vi "DiffDrivePoseEst_BiConsum_VisionCorrect.vi"(9 "Y":T2, 10 "U":T2, 11 "ExtraPassedData":variant) -> (0 "Error":bool, 3 "ExtraReturnedData":variant)   [LabVIEW 2019, in "Trajectory_Library.lvlib"]
doc: "Creates a new LINEAR SYSTEM data cluster with the specified values. \n\n\nInputs: \n - XXX -- XXX.\n\nOutputs:\n - XXX -- XXX."
uses:
  <vilib>/Analysis/Matrix/Datatypes/RealMatrix.ctl
  MatBuilder_Create.vi
  Trajectory_Library.lvlib
  DiffDrivePoseEst_BiFunc_H.vi
  AngleStats_AngleMean_BiFunc.vi
  AngleStats_AngleResidual_BiFunc.vi
  AngleStats_AngleAdd_BiFunc.vi
  <vilib>/Analysis/Matrix/NI_Matrix.lvlib
  MERWE_SCALED_SIGMA_PTS.ctl
  BiFun_Matrix_FUNC_TYPE.ctl
  UNSCENTED_KALMAN_FILTER.ctl
panel:
  in  "Cluster":T5
  # "State Estimate <Statess,1>"
  # "<States, States>"
  # "<States, ?>"
  # "<Statess,  States>"
  # "<Outputs, Outputs>"
  # "<?, 1>"
  # "<?, 1>"
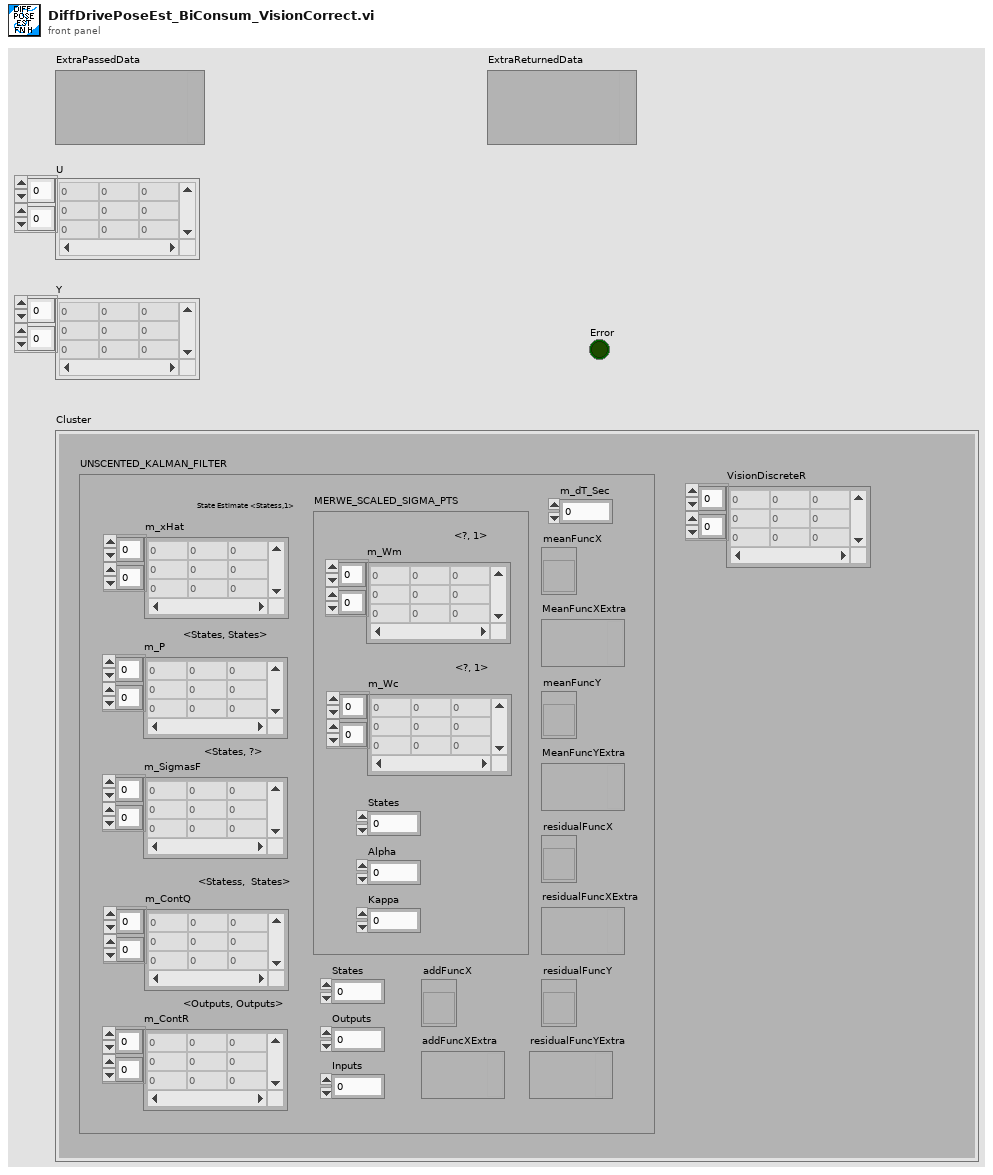
[diagram p1: front panel]
types:
  T1 = typedef "Trajectory_Library.lvlib/UNSCENTED_KALMAN_FILTER.ctl" = cluster{"m_P":T2, "m_xHat":T2, "States":i32, "Outputs":i32, "m_ContR":T2, "m_ContQ":T2, "m_SigmasF":T2, "m_dT_Sec":dbl, "MERWE_SCALED_SIGMA_PTS":T3, "meanFuncX":T4, "meanFuncY":T4, "residualFuncX":T4, "residualFuncY":T4, "addFuncX":T4, "addFuncXExtra":variant, "residualFuncYExtra":variant, "residualFuncXExtra":variant, "MeanFuncYExtra":variant, "MeanFuncXExtra":variant, "Inputs":i32}
  T2 = typedef "NI_Matrix.lvlib/RealMatrix.ctl" = dbl[][]
  T3 = typedef "Trajectory_Library.lvlib/MERWE_SCALED_SIGMA_PTS.ctl" = cluster{"m_Wm":T2, "States":i32, "Alpha":dbl, "m_Wc":T2, "Kappa":i32}
  T4 = typedef "Trajectory_Library.lvlib/BiFun_Matrix_FUNC_TYPE.ctl" = refnum<vi>
  T5 = cluster{"UNSCENTED_KALMAN_FILTER":T1, "VisionDiscreteR":T2}
  T6 = typedef "Trajectory_Library.lvlib/UNSCENTED_KALMAN_CORRECT_FUNC_GROUP.ctl" = cluster{"H_Func":T4, "meanFuncY":T4, "residualFuncY":T4, "residualFuncX":T4, "addFuncX":T4, "H_FuncExtra":variant, "MeanFuncYExtra":variant, "residualFuncYExtra":variant, "residualFuncXExtra":variant, "addFuncXExtra":variant}
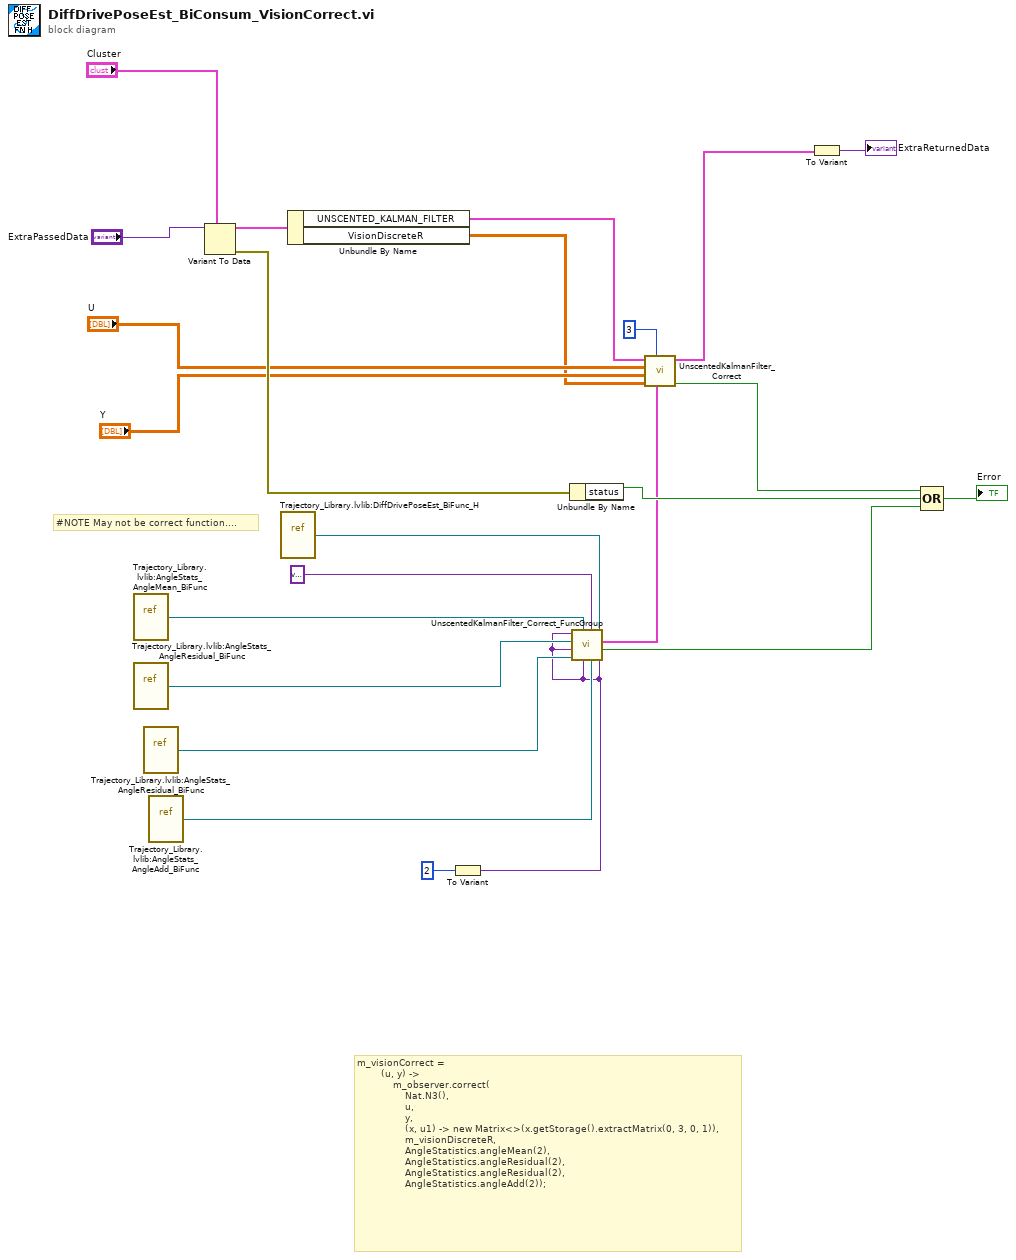
[diagram p0: block diagram]
diagram:
  # "#NOTE May not be correct function...."
  # "m_visionCorrect =\n        (u, y) ->\n            m_observer.correct(\n                Nat.N3(),\n                u,\n                y,\n                (x, u1) -> new Matrix<>(x.getStorage().extractMatrix(0, 3, 0, 1)),\n                m_visionDiscreteR,\n                AngleStatistics.angleMean(2),\n                AngleStatistics.angleResidual(2),\n                AngleStatistics.angleResidual(2),\n                AngleStatistics.angleAdd(2));"
  n1 = vi-ref "Trajectory_Library.lvlib:AngleStats_AngleMean_BiFunc.vi"() -> (w4:refnum<vi>)
  n2 = vi-ref "Trajectory_Library.lvlib:AngleStats_AngleResidual_BiFunc.vi"() -> (w5:refnum<vi>)
  n3 = vi-ref "Trajectory_Library.lvlib:AngleStats_AngleResidual_BiFunc.vi"() -> (w6:refnum<vi>)
  n4 = vi-ref "Trajectory_Library.lvlib:AngleStats_AngleAdd_BiFunc.vi"() -> (w7:refnum<vi>)
  n5 = Variant To Data(type="Cluster", Variant="ExtraPassedData") -> (data=w22:T5, error out=w17:errorcluster)  [unwired: 1 in]
  n6 = vi-ref "Trajectory_Library.lvlib:DiffDrivePoseEst_BiFunc_H.vi"() -> (w21:refnum<vi>)
  n7 = Unbundle By Name(w22) -> ("UNSCENTED_KALMAN_FILTER"=w19:T1, "VisionDiscreteR"=w11:T2)
  n8 = To Variant(anything=2) -> (Variant=w1:variant)
  n9 = Unbundle By Name(w17) -> ("status"=w16:bool)
  n10 = call "UnscentedKalmanFilter_Correct_FuncGroup.vi"("addFuncXExtra"=w1, "H_Func"=w21, "AddFuncX"=w7, "H_FuncExtra"=variant ("F_Func_ExtraData"), "residualFuncXExtra"=w1, "MeanFuncY"=w4, "ResidualFuncX"=w6, "residualFuncYExtra"=w1, "ResidualFuncY"=w5, "MeanFuncYExtra"=w1) -> ("Error"=w3:bool, "UNSCENTED_KALMAN_CORRECT_FUNC_GROUP"=w12:T6)
  n11 = call "UnscentedKalmanFilter_Correct.vi"("UNSCENTED_KALMAN_CORRECT_FUNC_GROUP"=w12, "Rows"=3, "R"=w11, "Y"="Y", "U"="U", "in UnscentedKalmanFiilter"=w19) -> ("Error"=w15:bool, "out UnscentedKalmanFiilter"=w8:T1)  [unwired: 4 in]
  n12 = To Variant(anything=w8) -> (Variant=→"ExtraReturnedData":variant)
  n13 = Compound Arithmetic op=OR(w15, w16, w3) -> (→"Error":bool)
